vi "GetAllAvailableRecords.vi"(8 "error in (no error)":errorcluster, 11 "Scope5785_six_channel":refnum<class "Scope5782_six_channel.lvclass">) -> (0 "error out":errorcluster, 2 "Available records":i32, 3 "Scope5785_six_channel out":refnum<class "Scope5782_six_channel.lvclass">)   [LabVIEW 2025, in "Scope5782_six_channel.lvclass"]
uses:
  Scope5782_six_channel.lvclass
  Scope5782_six_channel.lvclass/Scope5782_six_channel.ctl
  FpgaRef/FpgaRef5761/FpgaRef5761.lvclass
  FpgaRef/FpgaRefx410/FpgaRefx410.lvclass
  FpgaRef/FpgaRefBase/FpgaRefBase.lvclass
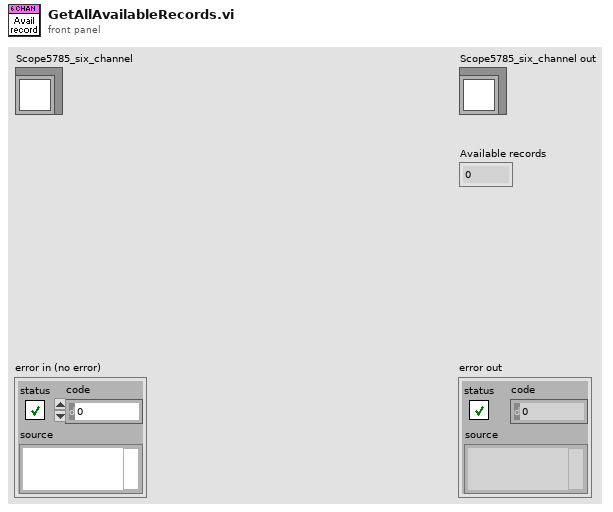
[diagram p1: front panel]
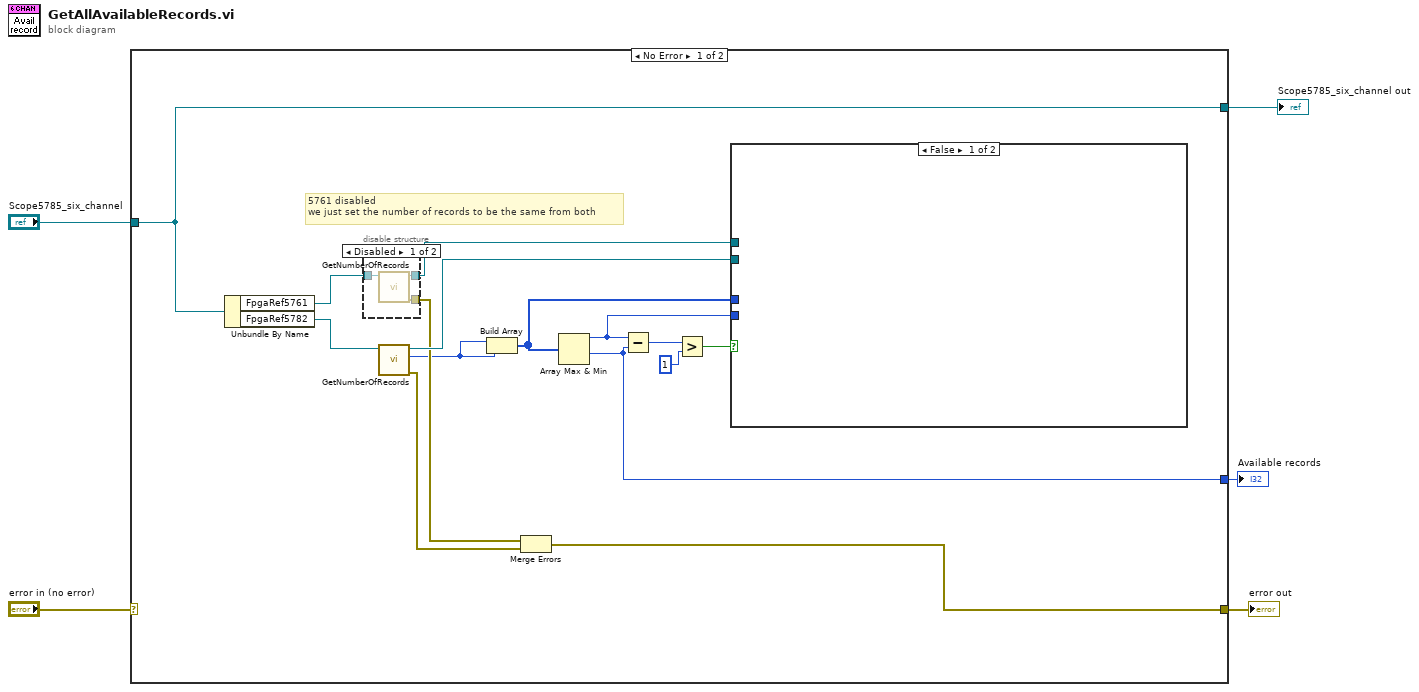
[diagram p0: block diagram]
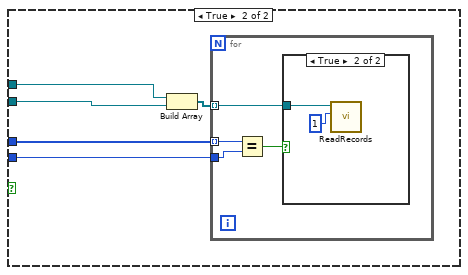
[diagram p3: hidden frame]
diagram:
  n1 = case shown="No Error" "error in (no error)" {
    selector: "error in (no error)" -> [_ w37]
    tunnel: [w7 w37] -> w4
    tunnel: [w10 w36] -> w2
    tunnel: "Scope5785_six_channel" -> [w10 w36]
    tunnel: [w13 _] -> w1
    frame No Error {
      # "5761 disabled\nwe just set the number of records to be the same from both"
      n2 = Unbundle By Name(w10) -> ("FpgaRef5761"=w20:refnum<class "FpgaRef5761.lvclass">, "FpgaRef5782"=w19:refnum<class "FpgaRefx410.lvclass">)
      n3 = disable-structure shown="Disabled" {
        disable-tunnel: w20 -> [w23 w24]
        disable-tunnel: [w22 w24] -> w12
        disable-tunnel: [w21 _] -> w9
        frame Disabled {
          n4 = call-dynamic "GetNumberOfRecords.vi"("FpgaRef5761 In"=w23) -> ("error out"=w21:errorcluster, "FpgaRef5761 Out"=w22:refnum<class "FpgaRef5761.lvclass">)  [unwired: 8 in, 1 out]
        }
        frame Enabled {
        }
      }
      n5 = call-dynamic "GetNumberOfRecords.vi"("FpgaRef5782 in"=w19) -> ("error out"=w8:errorcluster, "number of records"=w6:i32, "FpgaRef5782 out"=w11:refnum<class "FpgaRefx410.lvclass">)  [unwired: 8 in]
      n6 = Build Array(w6, w6) -> (w15:i32[])
      n7 = Merge Errors(w9, w8) -> (w7:errorcluster)
      n8 = Array Max & Min(array=w15) -> (max value=w14:i32, min value=w13:i32)  [unwired: 2 out]
      n9 = Subtract(x=w14, y=w13) -> (x-y=w18:i32)
      n10 = Greater?(x=w18, y=1) -> (0:w16:bool)
      n11 = case shown="False" w16 {
        tunnel: w15 -> [_ w28]
        tunnel: w14 -> [_ w27]
        tunnel: w12 -> [_ w26]
        tunnel: w11 -> [_ w25]
        frame False {
        }
        frame True {
          n12 = Build Array(w26, w25) -> (w29:refnum<class "FpgaRefBase.lvclass">[])
          n13 = for {
            tunnel: w29 -> [w31] mode=indexing
            tunnel: w28 -> [w33] mode=indexing
            tunnel: w27 -> [w32]
            n14 = Equal?(x=w33, y=w32) -> (x = y?=w30:bool)
            n15 = case shown="True" w30 {
              tunnel: w31 -> [_ w35]
              frame False {
              }
              frame True {
                n16 = call-dynamic "ReadRecords.vi"("Num records to read"=1, "FpgaRefBase in"=w35) -> ()  [unwired: 7 in, 3 out]
              }
            }
          }
        }
      }
    }
    frame Error {
    }
  }
  "error out" <- w4
  "Scope5785_six_channel out" <- w2
  "Available records" <- w1
